vi "Calculate conductance ITX.vi"(0 "File or Folder Path":path=path "P:/expt/Leiden MNK/SA02836H.20170110/47", 5 "single ended?":bool=TRUE, 7 "index":T2={"N1"=18, "N2"=19, "N3"=4, "N4"=5, "V1"=8, "V2"=10, "V3"=10, "V4"=13, "CURRENT"=12, "Vsg"=1}, 9 "offset":i32, 11 "length":i32=1000) -> (3 "N Array":T1(array[cluster])=[{"N1"=191.996, "N2"=144.795, "N3"=0.00010057503022848991, "N4"=-1.0338940453395174e-05}, {"N1"=191.996, "N2"=147.003, "N3"=0.00010066534958225373, "N4"=-1.0380780420219314e-05}, {"N1"=191.996, "N2"=149.362, "N3"=0.00010045742974572892, "N4"=-1.0407899416737152e-05}, {"N1"=191.996, "N2"=151.724, "N3"=0.0001005426468584359, "N4"=-1.041982763249689e-05}, {"N1"=191.996, "N2"=154.337, "N3"=0.00010054163078601866, "N4"=-1.0324258520933678e-05}, {"N1"=191.996, "N2"=156.886, "N3"=0.00010056662242594223, "N4"=-1.038386753752895e-05}, {"N1"=191.996, "N2"=159.496, "N3"=0.0001006132221954114, "N4"=-1.0237620457409125e-05}, {"N1"=191.996, "N2"=161.991, "N3"=0.00010051966642671815, "N4"=-1.0219524315805733e-05}, {"N1"=191.996, "N2"=164.35, "N3"=0.00010054011068586918, "N4"=-1.0306705331260904e-05}, {"N1"=191.996, "N2"=166.841, "N3"=0.00010064457917184225, "N4"=-1.0165964089479782e-05}, {"N1"=191.996, "N2"=169.349, "N3"=0.00010053072958605225, "N4"=-1.0410678322353806e-05}, {"N1"=191.996, "N2"=172.005, "N3"=0.0001004938480593684, "N4"=-1.0388414744068434e-05}, {"N1"=191.996, "N2"=174.505, "N3"=0.00010066827534930882, "N4"=-1.0395636867591871e-05}, {"N1"=191.996, "N2"=177.006, "N3"=0.0001005048646735938, "N4"=-1.0223947706368497e-05}, {"N1"=191.996, "N2"=179.504, "N3"=0.00010058085140214634, "N4"=-1.0431970547534671e-05}, {"N1"=191.996, "N2"=181.84, "N3"=0.00010052922489490765, "N4"=-1.0355084186355676e-05}, {"N1"=191.996, "N2"=184.374, "N3"=0.00010058119857393249, "N4"=-1.0414147914325042e-05}, {"N1"=191.996, "N2"=187.017, "N3"=0.00010055623762781604, "N4"=-1.0471997511387608e-05}, {"N1"=191.996, "N2"=189.493, "N3"=0.00010061746471290358, "N4"=-1.0469366265831165e-05}, {"N1"=191.996, "N2"=192.044, "N3"=0.00010054215797227613, "N4"=-1.035195576109068e-05}, {"N1"=191.996, "N2"=194.506, "N3"=0.00010070522372706563, "N4"=-1.0337727806851342e-05}, {"N1"=191.996, "N2"=196.968, "N3"=0.00010065305882857154, "N4"=-1.0272321635940252e-05}, {"N1"=191.996, "N2"=199.515, "N3"=0.00010065777271444059, "N4"=-1.0350588285323707e-05}, {"N1"=191.996, "N2"=201.997, "N3"=0.00010058385854993672, "N4"=-1.0306678170450834e-05}, {"N1"=191.996, "N2"=204.265, "N3"=0.00010061221693842934, "N4"=-1.0065603355709244e-05}, {"N1"=191.996, "N2"=206.999, "N3"=0.0001005875811108127, "N4"=-1.0206305681344109e-05}, {"N1"=191.996, "N2"=209.539, "N3"=0.00010058820923197684, "N4"=-1.0493263333126373e-05}, {"N1"=191.996, "N2"=212.028, "N3"=0.00010061805295099033, "N4"=-1.0298862286088797e-05}, {"N1"=191.996, "N2"=214.443, "N3"=0.00010055810354804531, "N4"=-1.0563400445389847e-05}, {"N1"=191.996, "N2"=216.725, "N3"=0.00010053926676591393, "N4"=-1.038753898763444e-05}, {"N1"=191.996, "N2"=219.47, "N3"=0.00010058066546024038, "N4"=-1.03096656971029e-05}, {"N1"=191.996, "N2"=221.797, "N3"=0.000100521698263223, "N4"=-1.033180469731966e-05}, {"N1"=191.996, "N2"=224.497, "N3"=0.0001004795934350268, "N4"=-1.0405173181004657e-05}, {"N1"=191.996, "N2"=226.998, "N3"=0.00010059015791575789, "N4"=-1.033766826105032e-05}, {"N1"=191.996, "N2"=229.436, "N3"=0.00010060923714347418, "N4"=-1.0267885998498252e-05}, {"N1"=191.996, "N2"=231.634, "N3"=0.00010049651116289272, "N4"=-1.0430449385843277e-05}, {"N1"=191.996, "N2"=234.5, "N3"=0.00010055712089386373, "N4"=-1.0358131509413556e-05}, {"N1"=191.996, "N2"=236.999, "N3"=0.00010068379827598355, "N4"=-1.0302561579314388e-05}, {"N1"=191.996, "N2"=239.477, "N3"=0.00010047866336560874, "N4"=-1.0411909259862328e-05}, {"N1"=191.996, "N2"=241.853, "N3"=0.00010055343454259429, "N4"=-1.0243657310468301e-05}, {"N1"=191.996, "N2"=244.405, "N3"=0.00010058417717772568, "N4"=-1.0269493681777803e-05}, {"N1"=191.996, "N2"=246.91, "N3"=0.00010062819456533582, "N4"=-1.0272141148598907e-05}, {"N1"=191.996, "N2"=249.488, "N3"=0.00010056821029236928, "N4"=-1.0340020021854818e-05}, {"N1"=191.996, "N2"=251.704, "N3"=0.00010065759557074449, "N4"=-1.0329641383071122e-05}, {"N1"=191.996, "N2"=254.492, "N3"=0.00010057796952190451, "N4"=-1.0284612827778078e-05}, {"N1"=191.996, "N2"=256.799, "N3"=0.00010063577042569525, "N4"=-1.0329227866710886e-05}, {"N1"=189.506, "N2"=256.99, "N3"=0.00010053195853199196, "N4"=-1.0445442874501309e-05}, {"N1"=189.506, "N2"=254.642, "N3"=0.00010062373739047002, "N4"=-1.038267676413735e-05}, {"N1"=189.506, "N2"=252.252, "N3"=0.00010060901043629462, "N4"=-1.0423317753346132e-05}, {"N1"=189.506, "N2"=249.855, "N3"=0.00010050094587740504, "N4"=-1.0431223967160507e-05}, {"N1"=189.506, "N2"=246.999, "N3"=0.00010058974428219982, "N4"=-1.0340299277280957e-05}, {"N1"=189.506, "N2"=244.524, "N3"=0.00010055656468780623, "N4"=-1.053351676682195e-05}, {"N1"=189.506, "N2"=242.248, "N3"=0.00010055388255591169, "N4"=-1.0216325327280904e-05}, {"N1"=189.506, "N2"=240.113, "N3"=0.00010057451174382039, "N4"=-1.041060384291682e-05}, {"N1"=189.506, "N2"=236.998, "N3"=0.00010054319017101952, "N4"=-1.0348870506195839e-05}, {"N1"=189.506, "N2"=234.866, "N3"=0.00010050860466242158, "N4"=-1.0475965819222953e-05}, {"N1"=189.506, "N2"=231.979, "N3"=0.00010060735713010531, "N4"=-1.0374517256243438e-05}, {"N1"=189.506, "N2"=229.88, "N3"=0.00010049947613491992, "N4"=-1.0491154630192516e-05}, {"N1"=189.506, "N2"=227.267, "N3"=0.00010062560576095063, "N4"=-1.0555557528305423e-05}, {"N1"=189.506, "N2"=224.473, "N3"=0.00010054870210895435, "N4"=-1.0387256544361327e-05}, {"N1"=189.506, "N2"=222.338, "N3"=0.0001005705880949266, "N4"=-1.0359666369953541e-05}, {"N1"=189.506, "N2"=219.943, "N3"=0.00010052399645025834, "N4"=-1.0310144901537403e-05}, {"N1"=189.506, "N2"=217.359, "N3"=0.00010060901318214533, "N4"=-1.0430222257765288e-05}, {"N1"=189.506, "N2"=214.968, "N3"=0.0001005359008706473, "N4"=-1.0310194088582675e-05}, {"N1"=189.506, "N2"=212.385, "N3"=0.00010054874079276358, "N4"=-1.0350840870693861e-05}, {"N1"=189.506, "N2"=209.538, "N3"=0.00010052877064697572, "N4"=-1.0448750460944099e-05}, {"N1"=189.506, "N2"=207.267, "N3"=0.00010053680956204742, "N4"=-1.0355852855433731e-05}, {"N1"=189.506, "N2"=204.668, "N3"=0.00010057308714312922, "N4"=-1.0381850165958104e-05}, {"N1"=189.506, "N2"=201.992, "N3"=0.00010051465119619463, "N4"=-1.0253710037528991e-05}, {"N1"=189.506, "N2"=199.708, "N3"=0.00010054552600488515, "N4"=-1.0111514624342852e-05}, {"N1"=189.506, "N2"=197.028, "N3"=0.00010056463679786198, "N4"=-1.0131100186631911e-05}, {"N1"=189.506, "N2"=194.795, "N3"=0.00010052779216466223, "N4"=-1.0611826314801406e-05}, {"N1"=189.506, "N2"=192.336, "N3"=0.00010061170953168135, "N4"=-1.0313720182691726e-05}, {"N1"=189.506, "N2"=189.856, "N3"=0.00010049183044402859, "N4"=-1.0574827403736794e-05}, {"N1"=189.506, "N2"=187.38, "N3"=0.00010057831497383143, "N4"=-1.0526665896714861e-05}, {"N1"=189.506, "N2"=184.506, "N3"=0.0001005504195817918, "N4"=-1.0419727243247705e-05}, {"N1"=189.506, "N2"=182.041, "N3"=0.00010053309735838938, "N4"=-1.027504174089921e-05}, {"N1"=189.506, "N2"=179.521, "N3"=0.00010063619607854753, "N4"=-1.0259288158518756e-05}, {"N1"=189.506, "N2"=177.348, "N3"=0.00010056552179621183, "N4"=-1.0306944055227605e-05}, {"N1"=189.506, "N2"=174.768, "N3"=0.00010050767014227269, "N4"=-1.0363158516396958e-05}, {"N1"=189.506, "N2"=171.99, "N3"=0.00010049993887402406, "N4"=-1.0288583567424436e-05}], 4 "A vs D":cluster{dbl[], dbl[]}[](graph), 6 "Index, Wavenames":string[][](table)=[["0", "'time.SA02836H.20170110.000034'\n"], ["1", "'Vsg.SA02836H.20170110.000034'\n"], ["2", "'T.SA02836H.20170110.000034'\n"], ["3", "'B.SA02836H.20170110.000034'\n"], ["4", "'X0.SA02836H.20170110.000034'\n"], ["5", "'Y0.SA02836H.20170110.000034'\n"], ["6", "'X1.SA02836H.20170110.000034'\n"], ["7", "'Y1.SA02836H.20170110.000034'\n"], ["8", "'X2.SA02836H.20170110.000034'\n"], ["9", "'Y2.SA02836H.20170110.000034'\n"], ["10", "'X3.SA02836H.20170110.000034'\n"], ["11", "'Y3.SA02836H.20170110.000034'\n"], ["12", "'X4.SA02836H.20170110.000034'\n"], ["13", "'Y4.SA02836H.20170110.000034'\n"], ["14", "'X5.SA02836H.20170110.000034'\n"], ["15", "'Y5.SA02836H.20170110.000034'\n"], ["16", "'B_rate.SA02836H.20170110.000034'\n"], ["17", "'R4t(e2/h).SA02836H.20170110.000034'\n"], ["18", "'axis1.SA02836H.20170110.000034'\n"], ["19", "'axis2.SA02836H.20170110.000034'\n"], ["", ""]], 8 "Comments":string="IGOR\nX// Date: 2/20/2017 3:49 PM\nX// B=18T\nX// large axis: 192 -- 184.5, 2.5 deg steps\nX// small axis: 144.5 -- 257, 2.5 deg steps\nX// sweep Vsg: 50mV to 170mV, 250uV steps\nX// Vbg=0.45V\nX// T<50mK\nX// \nX// lockin settings: \nX// tc=0.3s\nX// order=4\nX// prefilters OFF\nX// \nX// 0: 1, voltage\nX// 1: 2, current, 100uV AC 240uV DC, 13 Hz\nX// 2: 3, voltage\nX// 3: 4, voltage\nX// 4: 5, current\nX// 5: 7, voltage\nX//  \nX// KH gain=100x, shunt resistor=50kOhm\nX// \nX// axis1=189.506000\nX// axis2=171.990000\n\n\n\n\n\n\n\n\n\n\n\n\n\n\n\n\n\n\n\n\n\n\n\n\n\n\n\n\n\n\n\n\n\n\n\n\n\n\n\n\n\n\nX \nX Display/R 'time.SA02836H.20170110.000034'\nX AppendToGraph 'Vsg.SA02836H.20170110.000034'\nX AppendToGraph 'T.SA02836H.20170110.000034'\nX AppendToGraph 'B.SA02836H.20170110.000034'\nX AppendToGraph 'X0.SA02836H.20170110.000034'\nX AppendToGraph 'Y0.SA02836H.20170110.000034'\nX AppendToGraph 'X1.SA02836H.20170110.000034'\nX AppendToGraph 'Y1.SA02836H.20170110.000034'\nX AppendToGraph 'X2.SA02836H.20170110.000034'\nX AppendToGraph 'Y2.SA02836H.20170110.000034'\nX AppendToGraph 'X3.SA02836H.20170110.000034'\nX AppendToGraph 'Y3.SA02836H.20170110.000034'\nX AppendToGraph 'X4.SA02836H.20170110.000034'\nX AppendToGraph 'Y4.SA02836H.20170110.000034'\nX AppendToGraph 'X5.SA02836H.20170110.000034'\nX AppendToGraph 'Y5.SA02836H.20170110.000034'\nX AppendToGraph 'B_rate.SA02836H.20170110.000034'\nX AppendToGraph 'R4t(e2/h).SA02836H.20170110.000034'\nX AppendToGraph 'axis1.SA02836H.20170110.000034'\nX AppendToGraph 'axis2.SA02836H.20170110.000034'\nX Label bottom \"x label\"\nX Label left \"y label\"\nX ModifyGraph rgb('time.SA02836H.20170110.000034')=(65280,0,0)\nX ModifyGraph rgb('Vsg.SA02836H.20170110.000034')=(65280,18432,0)\nX ModifyGraph rgb('T.SA02836H.20170110.000034')=(65280,35328,0)\nX ModifyGraph rgb('B.SA02836H.20170110.000034')=(65280,52224,0)\nX ModifyGraph rgb('X0.SA02836H.20170110.000034')=(60416,65280,0)\nX ModifyGraph rgb('Y0.SA02836H.20170110.000034')=(41984,65280,0)\nX ModifyGraph rgb('X1.SA02836H.20170110.000034')=(25088,65280,0)\nX ModifyGraph rgb('Y1.SA02836H.20170110.000034')=(8192,65280,0)\nX ModifyGraph rgb('X2.SA02836H.20170110.000034')=(0,65280,10240)\nX ModifyGraph rgb('Y2.SA02836H.20170110.000034')=(0,65280,28672)\nX ModifyGraph rgb('X3.SA02836H.20170110.000034')=(0,65280,45568)\nX ModifyGraph rgb('Y3.SA02836H.20170110.000034')=(0,65280,62464)\nX ModifyGraph rgb('X4.SA02836H.20170110.000034')=(0,50176,65280)\nX ModifyGraph rgb('Y4.SA02836H.20170110.000034')=(0,31744,65280)\nX ModifyGraph rgb('X5.SA02836H.20170110.000034')=(0,14848,65280)\nX ModifyGraph rgb('Y5.SA02836H.20170110.000034')=(2048,0,65280)\nX ModifyGraph rgb('B_rate.SA02836H.20170110.000034')=(20480,0,65280)\nX ModifyGraph rgb('R4t(e2/h).SA02836H.20170110.000034')=(38912,0,65280)\nX ModifyGraph rgb('axis1.SA02836H.20170110.000034')=(55808,0,65280)\nX ModifyGraph rgb('axis2.SA02836H.20170110.000034')=(65280,0,58368)\nX Legend/C/N=text0/J \"\\\\s('time.SA02836H.20170110.000034') time\\r\\\\s('Vsg.SA02836H.20170110.000034') Vsg\\r\\\\s('T.SA02836H.20170110.000034') T\\r\\\\s('B.SA02836H.20170110.000034') B\\r\\\\s('X0.SA02836H.20170110.000034') X0\\r\\\\s('Y0.SA02836H.20170110.000034') Y0\\r\\\\s('X1.SA02836H.20170110.000034') X1\\r\\\\s('Y1.SA02836H.20170110.000034') Y1\\r\\\\s('X2.SA02836H.20170110.000034') X2\\r\\\\s('Y2.SA02836H.20170110.000034') Y2\\r\\\\s('X3.SA02836H.20170110.000034') X3\\r\\\\s('Y3.SA02836H.20170110.000034') Y3\\r\\\\s('X4.SA02836H.20170110.000034') X4\\r\\\\s('Y4.SA02836H.20170110.000034') Y4\\r\\\\s('X5.SA02836H.20170110.000034') X5\\r\\\\s('Y5.SA02836H.20170110.000034') Y5\\r\\\\s('B_rate.SA02836H.20170110.000034') B_rate\\r\\\\s('R4t(e2/h).SA02836H.20170110.000034') R4t (e2/h)\\r\\\\s('axis1.SA02836H.20170110.000034') axis 1\\r\\\\s('axis2.SA02836H.20170110.000034') axis 2\"\nX ModifyGraph mirror(bottom)=1\nX ModifyGraph width=216\nX ModifyGraph height={Aspect,0.6}\nX ModifyGraph Log(bottom)=0\nX ModifyGraph Log(left)=0\nX \n")   [LabVIEW 2016]
uses:
  <vilib>/Utility/miscctls.llb/LVOffsetAndMultiplierTypeDef.ctl
  <vilib>/Analysis/NI_AALPro.lvlib
panel:
  out "A vs D diff":cluster{dbl[], dbl[]}[](graph)
  in  "Numeric":dbl=50.0
  in  "dy/dx vs x":bool=TRUE
  out "angle phi":dbl[](array[numeric])=[90.00000409114715, 90.00000404600523, 90.0000039925062, 90.00000393485637, 90.00000383275845, 90.00000379225543, 90.00000367766242, 90.00000361461817, 90.00000359312878, 90.00000349114927, 90.00000352224065, 90.00000346043615, 90.00000341323239, 90.00000330943048, 90.00000332977474, 90.00000326277288, 90.00000323628453, 90.00000320827124, 90.00000316555494, 90.00000308847648, 90.0000030451923, 90.00000298810302, 90.00000297243328, 90.0000029234551, 90.00000282337449, 90.0000028250293, 90.00000286924964, 90.00000278303499, 90.0000028223736, 90.00000274616285, 90.00000269148555, 90.00000266896669, 90.00000265559233, 90.00000260929507, 90.00000256414222, 90.00000258002162, 90.0000025308197, 90.00000249069954, 90.00000249108874, 90.00000242675647, 90.00000240747384, 90.00000238366341, 90.00000237462126, 90.00000235135259, 90.00000231545553, 90.00000230460853, 90.00000232880578, 90.00000233615648, 90.00000236752183, 90.00000239204782, 90.00000239861501, 90.00000246816694, 90.00000241633502, 90.00000248417896, 90.00000250190551, 90.00000255562162, 90.0000025623701, 90.00000261483767, 90.00000266113821, 90.0000026513031, 90.00000266965233, 90.00000268582218, 90.00000274940405, 90.00000274799322, 90.00000279237939, 90.0000028570918, 90.0000028627165, 90.00000290634686, 90.00000290850286, 90.00000290097098, 90.00000294612585, 90.00000312129605, 90.00000307239746, 90.00000319132911, 90.00000321877216, 90.0000032357018, 90.00000323397765, 90.00000327434626, 90.00000332986215, 90.00000339744831, 90.00000342748076]
  in  "e^2/h?":bool=TRUE
  in  "T=conductance\nF=resistance":bool=TRUE
  out "angle theta":dbl[](array[numeric])=[3.979781592245742e-05, 3.923525148650886e-05, 3.8535817310704016e-05, 3.7968082347300365e-05, 3.7324887158624575e-05, 3.6727579420033637e-05, 3.614330763786105e-05, 3.5553534729170675e-05, 3.505034386417848e-05, 3.456290490596515e-05, 3.401252157763598e-05, 3.347503480032623e-05, 3.3052733780554244e-05, 3.253282129605657e-05, 3.210434466738831e-05, 3.1675650595023693e-05, 3.1256457942296714e-05, 3.080708181495749e-05, 3.04230555923191e-05, 2.9996465991900285e-05, 2.9664813910527506e-05, 2.9278844614143605e-05, 2.8906425841285385e-05, 2.85302780835941e-05, 2.8221454473483897e-05, 2.7841892323532745e-05, 2.7504568876298417e-05, 2.7189756904348253e-05, 2.6867535564891757e-05, 2.657965468232256e-05, 2.6258019918388047e-05, 2.596729919687742e-05, 2.5644247500042603e-05, 2.5389613605084715e-05, 2.512458667494002e-05, 2.4858293451836762e-05, 2.4569290521129328e-05, 2.4340848301301122e-05, 2.403990087551123e-05, 2.3821442838564363e-05, 2.3579913823692036e-05, 2.3350900524947192e-05, 2.3095836284456867e-05, 2.2912847639044594e-05, 2.2643906942458915e-05, 2.2453377596639828e-05, 2.2413545002011955e-05, 2.264086628013591e-05, 2.2852035579448446e-05, 2.3046487105912263e-05, 2.33335673815276e-05, 2.3561968391426693e-05, 2.378270649956887e-05, 2.3999096465037315e-05, 2.430695809914132e-05, 2.4519167746311992e-05, 2.4848701613163618e-05, 2.5048702913721435e-05, 2.5368498378776492e-05, 2.5664629003759286e-05, 2.5916713476722578e-05, 2.6186788105952318e-05, 2.652051139503117e-05, 2.67960013091869e-05, 2.7125354816864744e-05, 2.7488447335136823e-05, 2.7791857235427556e-05, 2.8154931039059754e-05, 2.8511353384149216e-05, 2.8846287024066625e-05, 2.9244215323624077e-05, 2.9568614260134713e-05, 2.997164506780307e-05, 3.032697286357333e-05, 3.0754151769332044e-05, 3.1224538336453484e-05, 3.164189484793498e-05, 3.211896826305098e-05, 3.248968109847988e-05, 3.2950341640601424e-05, 3.3479983364170464e-05]
  in  "log scale?":bool
  in  "calculate Ey":bool=TRUE
  in  "background":enum16{"do nothing", "subtract", "divide"}(ring)
  in  "Background":cluster{dbl[], dbl[]}[](graph)
  in  "A offset":dbl format="%#_6p"
  out "E 2":dbl[][](graph)
  out "counter":i32=80
  out "Path":path=path "P:/expt/Leiden MNK/SA02836H.20170110/47/47 - Sweep axis 1,2 - 1/SA02836H.20170110.000034.itx"
  in  "file contains 2D data?":bool
  out "N":cluster{"N1":dbl, "N2":dbl, "N3":dbl, "N4":dbl}={"N1"=189.506, "N2"=171.99, "N3"=0.00010049993887402406, "N4"=-1.0288583567424436e-05} {"N4" format="%#_6p"; "N3" format="%#_6p"; "N2" format="%#_6p"; "N1" format="%#_20p"}
  in  "Ey":T3={"Offset"=0.0, "Multiplier"=1.0}
  in  "Ex":T3={"Offset"=0.0, "Multiplier"=1.0}
  in  "recolor traces?":bool
  out "C vs D":cluster{dbl[], dbl[]}[](graph)
  out "E":dbl[][](graph)
  in  "B x name":string="Vsg (V)"
  in  "A y name":string="Conductance (S)"
  in  "Ex name":string="Ex name"
  in  "Ez name":string="Ez name"
  in  "D x name":string="Vsg (V)"
  in  "C y name":string="Conductance (S)"
  in  "Ey name":string="Ey name"
  out "time":string[][](table)=[["2/19/2017", "7:43 PM"], ["2/19/2017", "7:56 PM"], ["2/19/2017", "8:09 PM"], ["2/19/2017", "8:22 PM"], ["2/19/2017", "8:34 PM"], ["2/19/2017", "8:47 PM"], ["2/19/2017", "9:01 PM"], ["2/19/2017", "9:15 PM"], ["2/19/2017", "9:28 PM"], ["2/19/2017", "9:40 PM"], ["2/19/2017", "9:52 PM"], ["2/19/2017", "10:05 PM"], ["2/19/2017", "10:19 PM"], ["2/19/2017", "10:33 PM"], ["2/19/2017", "10:49 PM"], ["2/19/2017", "11:02 PM"], ["2/19/2017", "11:15 PM"], ["2/19/2017", "11:29 PM"], ["2/19/2017", "11:42 PM"], ["2/19/2017", "11:57 PM"], ["2/20/2017", "12:11 AM"], ["2/20/2017", "12:25 AM"], ["2/20/2017", "12:41 AM"], ["2/20/2017", "12:55 AM"], ["2/20/2017", "1:08 AM"], ["2/20/2017", "1:22 AM"], ["2/20/2017", "1:36 AM"], ["2/20/2017", "1:50 AM"], ["2/20/2017", "2:03 AM"], ["2/20/2017", "2:16 AM"], ["2/20/2017", "2:33 AM"], ["2/20/2017", "2:46 AM"], ["2/20/2017", "3:01 AM"], ["2/20/2017", "3:22 AM"], ["2/20/2017", "5:13 AM"], ["2/20/2017", "5:25 AM"], ["2/20/2017", "5:38 AM"], ["2/20/2017", "6:10 AM"], ["2/20/2017", "6:22 AM"], ["2/20/2017", "6:35 AM"], ["2/20/2017", "6:47 AM"], ["2/20/2017", "7:00 AM"], ["2/20/2017", "7:13 AM"], ["2/20/2017", "7:26 AM"], ["2/20/2017", "7:39 AM"], ["2/20/2017", "7:51 AM"], ["2/20/2017", "8:09 AM"], ["2/20/2017", "8:22 AM"], ["2/20/2017", "8:35 AM"], ["2/20/2017", "8:48 AM"], ["2/20/2017", "9:01 AM"], ["2/20/2017", "9:14 AM"], ["2/20/2017", "9:27 AM"], ["2/20/2017", "9:40 AM"], ["2/20/2017", "9:57 AM"], ["2/20/2017", "10:10 AM"], ["2/20/2017", "10:24 AM"], ["2/20/2017", "10:37 AM"], ["2/20/2017", "10:50 AM"], ["2/20/2017", "11:08 AM"], ["2/20/2017", "11:21 AM"], ["2/20/2017", "11:35 AM"], ["2/20/2017", "11:48 AM"], ["2/20/2017", "12:01 PM"], ["2/20/2017", "12:15 PM"], ["2/20/2017", "12:29 PM"], ["2/20/2017", "12:42 PM"], ["2/20/2017", "12:55 PM"], ["2/20/2017", "1:09 PM"], ["2/20/2017", "1:21 PM"], ["2/20/2017", "1:37 PM"], ["2/20/2017", "1:50 PM"], ["2/20/2017", "2:03 PM"], ["2/20/2017", "2:16 PM"], ["2/20/2017", "2:29 PM"], ["2/20/2017", "2:43 PM"], ["2/20/2017", "2:56 PM"], ["2/20/2017", "3:10 PM"], ["2/20/2017", "3:23 PM"], ["2/20/2017", "3:36 PM"], ["2/20/2017", "3:49 PM"]]
  in  "B is time?":bool
  in  "D  is time?":bool
  in  "Generate Folder Index File?":bool
  in  "pattern":string="*.itx"
  in  "Use Folder Index File?":bool
  # "CURRENT/(V1-V2)"
  # "CURRENT/(V3-V4)"
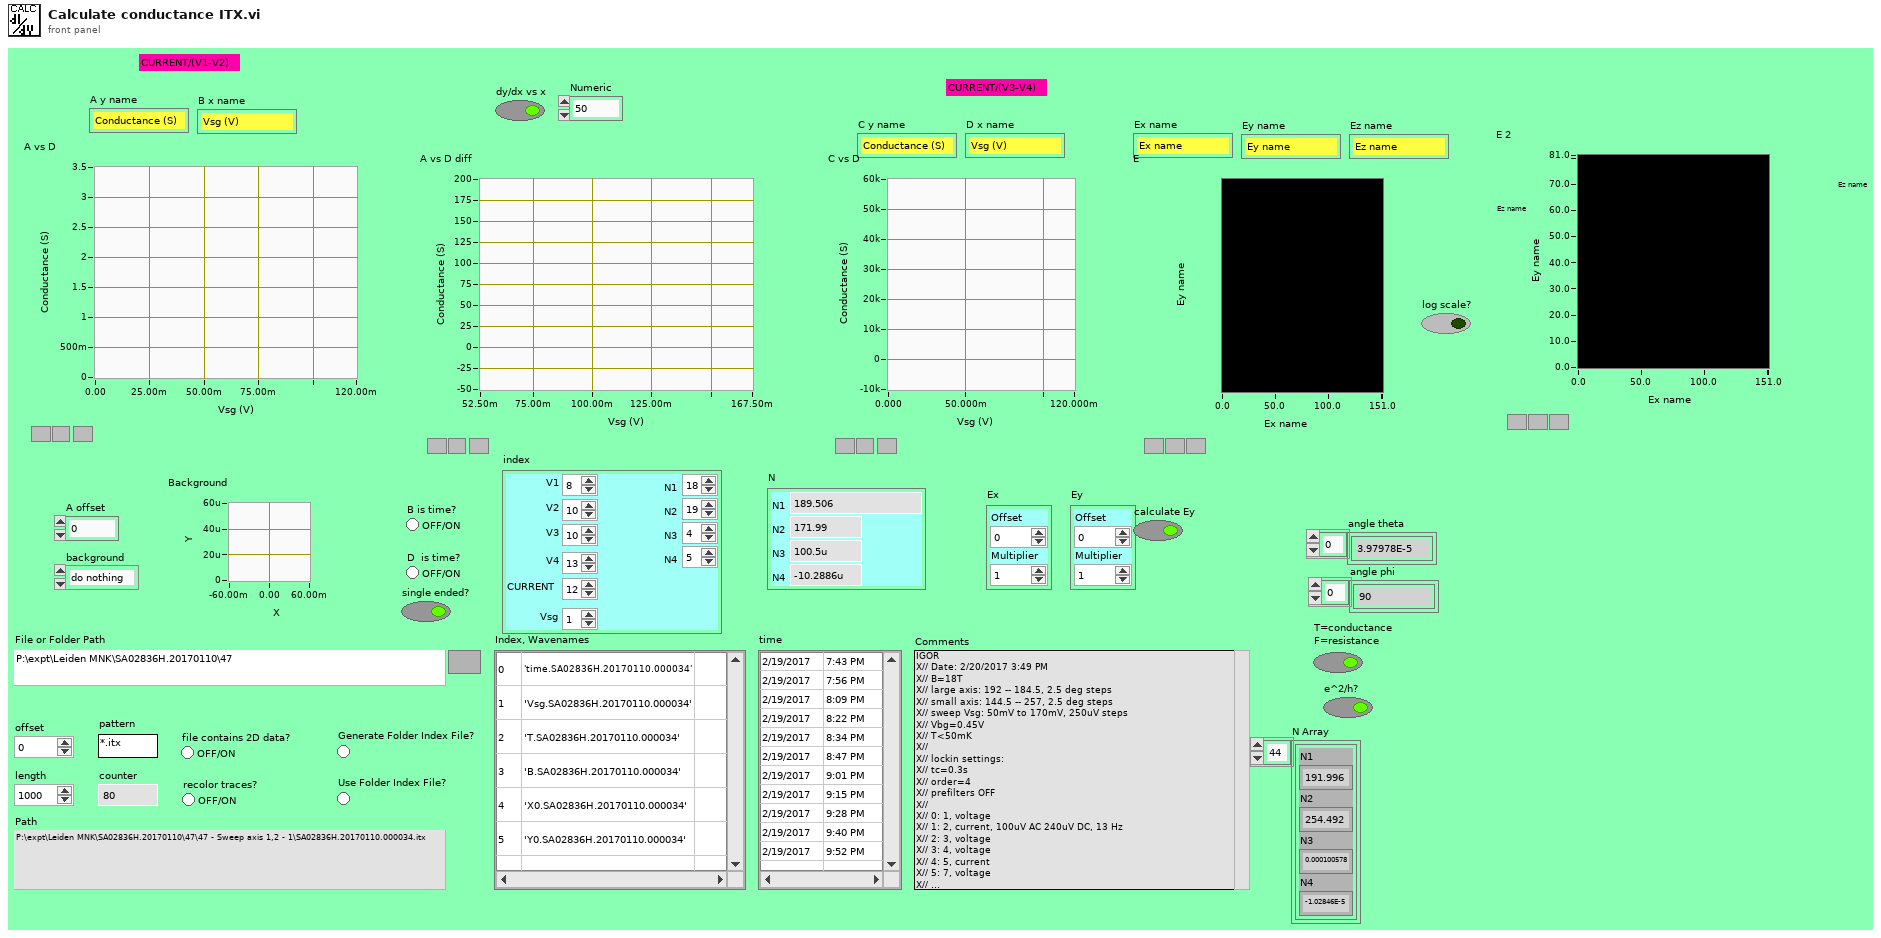
[diagram p1: front panel]
types:
  T1 = cluster{"N1":dbl, "N2":dbl, "N3":dbl, "N4":dbl}[]
  T2 = cluster{"N1":i32, "N2":i32, "N3":i32, "N4":i32, "V1":i32, "V2":i32, "V3":i32, "V4":i32, "CURRENT":i32, "Vsg":i32}
  T3 = typedef "LVOffsetAndMultiplierTypeDef.ctl" = cluster{"Offset":dbl, "Multiplier":dbl}
  T4 = cluster{"Decimated Array":dbl[], "Decimated Array":dbl[]}
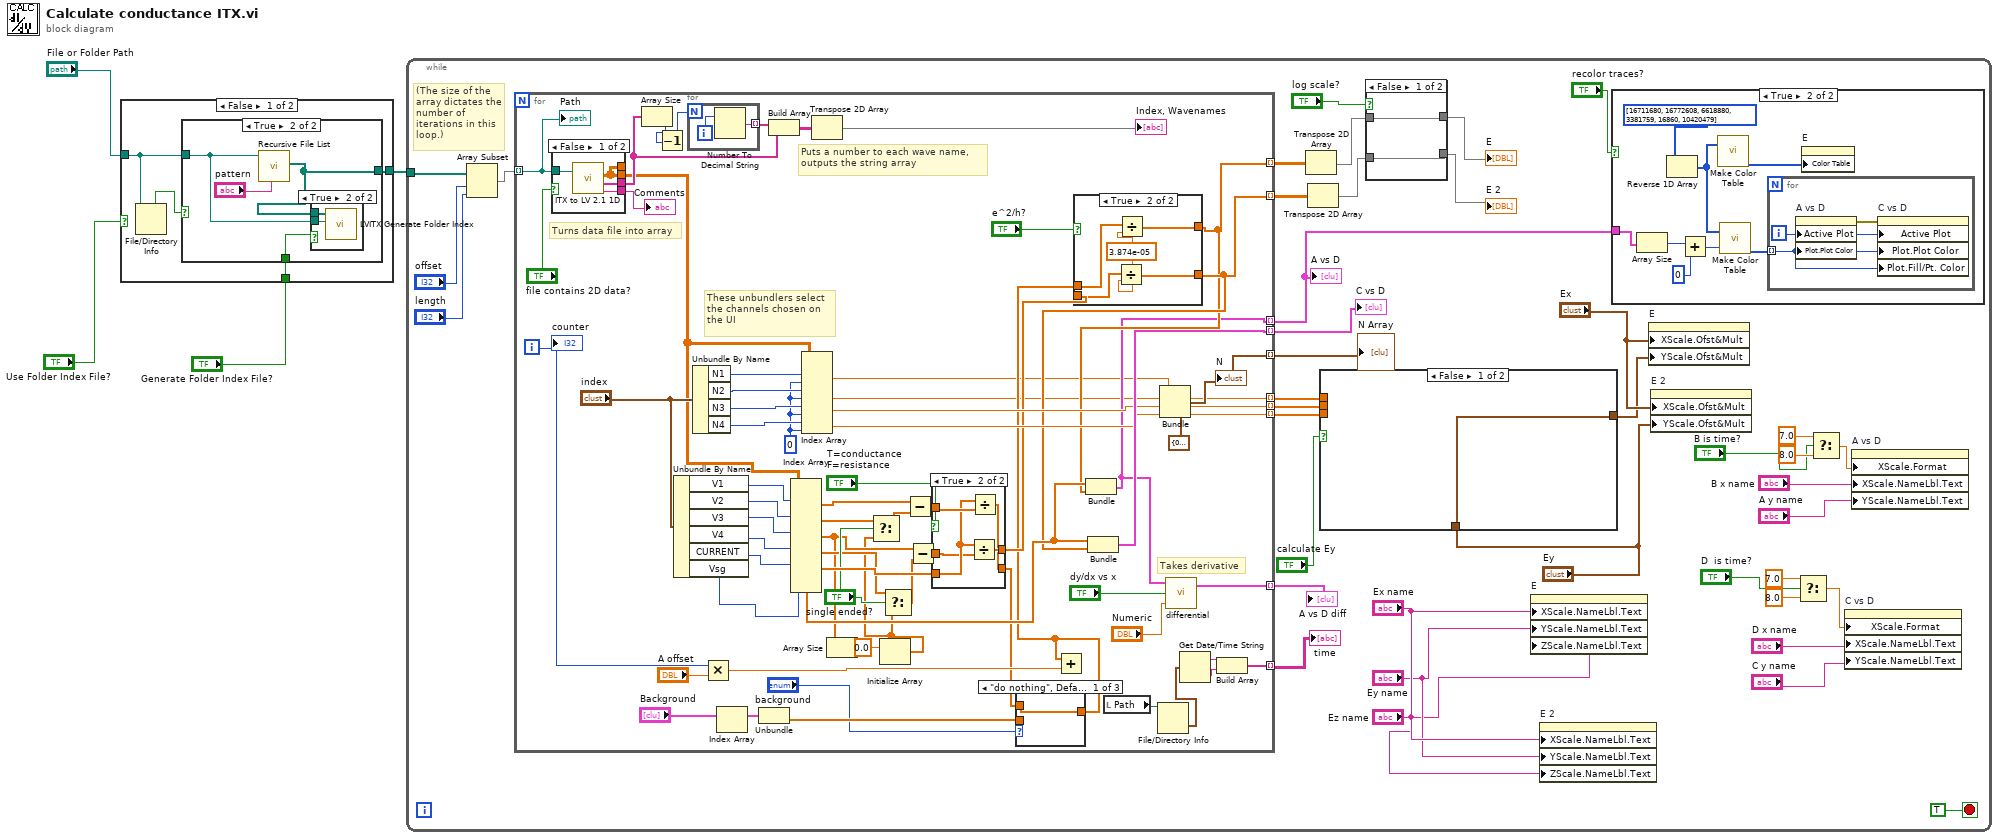
[diagram p0: block diagram]
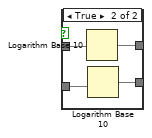
[diagram p2: hidden frame]
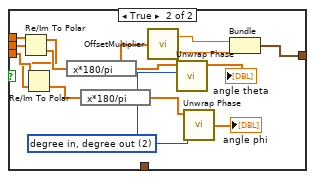
[diagram p3: hidden frame]
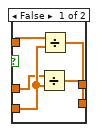
[diagram p6: hidden frame]
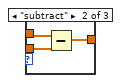
[diagram p7: hidden frame]
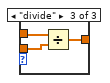
[diagram p8: hidden frame]
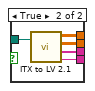
[diagram p9: hidden frame]
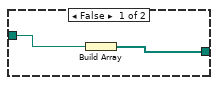
[diagram p10: hidden frame]
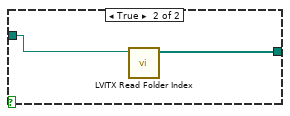
[diagram p12: hidden frame]
diagram:
  n1 = case shown="False" "Use Folder Index File?" {
    tunnel: [w6 w17] -> w2
    tunnel: "File or Folder Path" -> [w8 w18]
    tunnel: "Generate Folder Index File?" -> [w5 _]
    frame False {
      n2 = File/Directory Info(path=w8) -> (directory=w7:bool)  [unwired: 1 in, 6 out]
      n3 = case shown="True" w7 {
        tunnel: [w10 w13] -> w6
        tunnel: w8 -> [w9 w12]
        tunnel: w5 -> [_ w11]
        frame False {
          n4 = Build Array(w9) -> (w10:path[])
        }
        frame True {
          n5 = call <vilib>:"Recursive File List.vi"("pattern"="pattern", "Folder Path"=w12) -> ("All Files in Dir"=w13:path[])  [unwired: 5 in, 4 out]
          n6 = case shown="True" w11 {
            tunnel: w13 -> [_ w16]
            tunnel: w12 -> [_ w15]
            frame False {
            }
            frame True {
              n7 = call <userlib>:"LVITX Generate Folder Index.vi"("File or Folder Path"=w15, "All Files in Dir"=w16) -> ()  [unwired: 10 in]
            }
          }
        }
      }
    }
    frame True {
      n8 = call <userlib>:"LVITX Read Folder Index.vi"("File or Folder Path"=w18) -> ("Array"=w17:path[])  [unwired: 10 in]
    }
  }
  n9 = while {
    tunnel: w2 -> [w50]
    stop <- TRUE stop-if-true
    # "(The size of the array dictates the number of\niterations in this loop.)"
    n10 = Array Subset(array=w50, index="offset", length="length") -> (w49:path[])
    n11 = for {
      tunnel: w49 -> [w156] mode=indexing
      tunnel: [w156] -> _ mode=indexing
      tunnel: [w139] -> w53 mode=indexing
      tunnel: [w97] -> w39 mode=indexing
      tunnel: [w126] -> w40 mode=indexing
      tunnel: [w108] -> w38 mode=indexing
      tunnel: [w109] -> w37 mode=indexing
      tunnel: [w91] -> w31 mode=indexing
      tunnel: [w115] -> w30 mode=indexing
      tunnel: [w114] -> w29 mode=indexing
      tunnel: [w107] -> w20 mode=indexing
      tunnel: [w94] -> w19 mode=indexing
      i -> [w123]
      w137 = 0 ("disabled index (col)")
      # "Takes derivative"
      # "These unbundlers select\nthe channels chosen on\nthe UI"
      # "Puts a number to each wave name,\noutputs the string array"
      # "Turns data file into array"
      n12 = case shown="False" "file contains 2D data?" {
        tunnel: [w186 w189] -> w93
        tunnel: [w184 w190] -> w131
        tunnel: w156 -> [w185 w191]
        tunnel: [w183 w188] -> w149
        tunnel: [w184 w187] -> _
        frame False {
          n13 = call <userlib>:"ITX to LV 2.1 1D.vi"("file (use dialog)"=w185) -> ("1D arrays"=w184:dbl[][], "wave names"=w183:string[], "Notes"=w186:string)  [unwired: 2 in]
        }
        frame True {
          n14 = call <userlib>:"ITX to LV 2.1.vi"("file (use dialog)"=w191) -> ("2D array"=w187:dbl[][], "1D arrays"=w190:dbl[][], "wave names"=w188:string[], "Notes"=w189:string)  [unwired: 1 in]
        }
      }
      "Comments" <- w93
      n15 = Array Size(array=w149) -> (size(s)=w152:i32)
      n16 = Decrement(x=w152) -> (x-1=w151:i32)
      n17 = Unbundle By Name("index") -> ("V1"=w136:i32, "V2"=w135:i32, "V3"=w134:i32, "V4"=w133:i32, "CURRENT"=w130:i32, "Vsg"=w125:i32)
      n18 = for {
        N: w151 -> [_]
        tunnel: [w181] -> w154 mode=indexing
        i -> [w182]
        n19 = Number To Decimal String(number=w182) -> (decimal integer string=w181:string)  [unwired: 1 in]
      }
      n20 = Unbundle By Name("index") -> ("N1"=w144:i32, "N2"=w145:i32, "N3"=w146:i32, "N4"=w147:i32)
      n21 = Multiply(x=w123, y="A offset") -> (x*y=w121:dbl)
      n22 = Index Array(array="Background") -> (element=w117:cluster{dbl[], dbl[]})  [unwired: 1 in]
      n23 = Unbundle(w117) -> (w118:dbl[])  [unwired: 1 out]
      n24 = Build Array(w154, w149) -> (w150:string[][])
      n25 = Index Array(array=w131, index (row) #1=w136, index (row) #2=w135, index (row) #3=w134, index (row) #4=w133, index (row) #5=w130, index (row) #6=w125) -> (element #1=w132:dbl[], element #2=w105:dbl[], element #3=w101:dbl[], element #4=w103:dbl[], element #5=w128:dbl[], element #6=w124:dbl[])  [unwired: 6 in]
      n26 = Index Array(array=w131, index (row) #1=w144, index (col) #1=w137, index (row) #2=w145, index (col) #2=w137, index (row) #3=w146, index (col) #3=w137, index (row) #4=w147, index (col) #4=w137) -> (element #1=w92:dbl, element #2=w91:dbl, element #3=w115:dbl, element #4=w114:dbl)
      n27 = Transpose 2D Array(2D array=w150) -> (transposed array=→"Index, Wavenames":string[][])
      n28 = Array Size(array=w101) -> (size(s)=w99:i32)
      n29 = Initialize Array(0.0 ("element"), w99) -> (w98:dbl[])
      n30 = Select(t=w105, s="single ended?", f=w98) -> (s? t:f=w104:dbl[])
      n31 = Select(t=w103, s="single ended?", f=w98) -> (s? t:f=w102:dbl[])
      n32 = Subtract(x=w132, y=w104) -> (x-y=w129:dbl[])
      n33 = Subtract(x=w101, y=w102) -> (x-y=w127:dbl[])
      n34 = case shown="True" "T=conductance\nF=resistance" {
        tunnel: w129 -> [w168 w173]
        tunnel: w128 -> [w166 w172]
        tunnel: w127 -> [w165 w171]
        tunnel: [w164 w170] -> w112
        tunnel: [w167 w169] -> w120
        frame False {
          n35 = Divide(x=w165, y=w166) -> (x/y=w164:dbl[])
          n36 = Divide(x=w168, y=w166) -> (x/y=w167:dbl[])
        }
        frame True {
          n37 = Divide(x=w172, y=w171) -> (x/y=w170:dbl[])
          n38 = Divide(x=w172, y=w173) -> (x/y=w169:dbl[])
        }
      }
      n39 = case shown="\"do nothing\", Default" "background" {
        tunnel: w120 -> [w174 w177 w180]
        tunnel: [w174 w176 w178] -> w111
        tunnel: w118 -> [_ w175 w179]
        frame "do nothing", Default {
        }
        frame "subtract" {
          n40 = Subtract(x=w177, y=w175) -> (x-y=w176:dbl[])
        }
        frame "divide" {
          n41 = Divide(x=w180, y=w179) -> (x/y=w178:dbl[])
        }
      }
      n42 = Add(x=w111, y=w121) -> ()  [unwired: 1 out]
      n43 = case shown="True" "e^2/h?" {
        tunnel: w112 -> [w157 w161]
        tunnel: w111 -> [w158 w163]
        tunnel: [w158 w162] -> w108
        tunnel: [w157 w160] -> w109
        frame False {
        }
        frame True {
          w159 = 3.874e-05
          n44 = Divide(x=w161, y=w159) -> (x/y=w160:dbl[])
          n45 = Divide(x=w163, y=w159) -> (x/y=w162:dbl[])
        }
      }
      n46 = Bundle("1D arrays"=w124, w108) -> (w97:cluster{"1D arrays":dbl[], dbl[]})  [unwired: 1 in]
      n47 = Bundle("1D arrays"=w124, w109) -> (w126:cluster{"1D arrays":dbl[], dbl[]})  [unwired: 1 in]
      n48 = local read "Path"() -> (w143:path)
      n49 = File/Directory Info(path=w143) -> (last mod=w142:timestamp)  [unwired: 1 in, 6 out]
      n50 = Bundle(cluster=cluster{"N1":dbl, "N2":dbl, "N3":dbl, "N4":dbl} {"N1"=0.0, "N2"=0.0, "N3"=0.0, "N4"=0.0}, "N1"=w92, "N2"=w91, "N3"=w115, "N4"=w114) -> (w107:cluster{"N1":dbl, "N2":dbl, "N3":dbl, "N4":dbl})
      "N" <- w107
      n51 = call <userlib>:"differential.vi"("Numeric"="Numeric", "dy/dx vs x"="dy/dx vs x", "A vs B 2"=w97) -> ("A vs B 3"=w94:T4)  [unwired: 1 in]
      n52 = Get Date/Time String(seconds (now)=w142) -> (date string=w141:string, time string=w140:string)  [unwired: 2 in]
      n53 = Build Array(w141, w140) -> (w139:string[])
      "counter" <- w123
      "Path" <- w156
    }
    "A vs D" <- w39
    "C vs D" <- w40
    "time" <- w53
    "N Array" <- w20
    "A vs D diff" <- w19
    n54 = Transpose 2D Array(2D array=w38) -> (transposed array=w24:dbl[][])
    n55 = Transpose 2D Array(2D array=w37) -> (transposed array=w22:dbl[][])
    n56 = case shown="False" "calculate Ey" {
      tunnel: w31 -> [_ w79]
      tunnel: w30 -> [_ w78]
      tunnel: w29 -> [_ w67]
      tunnel: [w65 w74] -> w28
      tunnel: "Ey" -> [w65 _]
      frame False {
      }
      frame True {
        w70 = 2 items=["radian in, radian out", "radian in, degree out", "degree in, degree out", "degree in, radian out"] ("phase unit")
        n57 = Re/Im To Polar(2:w78, 3:w79) -> (0:w77:dbl[], 1:w66:dbl[])
        n58 = Re/Im To Polar(2:w66, 3:w67) -> (0:w68:dbl[])  [unwired: 1 out]
        n59 = expression code="x*180/pi"(w77) -> (w73:dbl[])
        n60 = expression code="x*180/pi"(w68) -> (w71:dbl[])
        n61 = call <userlib>:"OffsetMultiplier.vi"("Array"=w73) -> ("Offset"=w76:dbl, "Multiplier"=w75:dbl)
        n62 = call <vilib>:"Unwrap Phase.vi"("phase unit"=w70, "Phase"=w73) -> ("Unwrapped Phase"=→"angle theta":dbl[])  [unwired: 8 in, 1 out]
        n63 = call <vilib>:"Unwrap Phase.vi"("phase unit"=w70, "Phase"=w71) -> ("Unwrapped Phase"=→"angle phi":dbl[])  [unwired: 8 in, 1 out]
        n64 = Bundle("Offset"=w76, "Multiplier"=w75) -> (w74:cluster{"Offset":dbl, "Multiplier":dbl})  [unwired: 1 in]
      }
    }
    n65 = case shown="False" "log scale?" {
      tunnel: w24 -> [w60 w64]
      tunnel: [w60 w63] -> w23
      tunnel: w22 -> [w59 w62]
      tunnel: [w59 w61] -> w21
      frame False {
      }
      frame True {
        n66 = Logarithm Base 10(1:w64) -> (0:w63:dbl[][])
        n67 = Logarithm Base 10(1:w62) -> (0:w61:dbl[][])
      }
    }
    "E" <- w23
    "E 2" <- w21
    n68 = property on="E" class="IntGraph (strict)"("XScale.NameLbl.Text"="Ex name", "YScale.NameLbl.Text"="Ey name", "ZScale.NameLbl.Text"="Ez name") -> ()  [unwired: 2 in, 2 out]
    n69 = property on="E 2" class="IntGraph (strict)"("XScale.NameLbl.Text"="Ex name", "YScale.NameLbl.Text"="Ey name", "ZScale.NameLbl.Text"="Ez name") -> ()  [unwired: 2 in, 2 out]
    n70 = case shown="True" "recolor traces?" {
      tunnel: w39 -> [_ w80]
      frame False {
      }
      frame True {
        n71 = Array Size(array=w80) -> (size(s)=w83:i32)
        n72 = Reverse 1D Array(array=u32[] [16711680, 16772608, 6618880, 3381759, 16860, 10420479] ("color scale")) -> (reversed array=w82:u32[])
        n73 = Add(x=w83, y=0 ("x")) -> (x+y=w87:i32)
        n74 = call <userlib>:"Make Color Table.vi"("Array"=w82) -> ("Color Tbl"=w85:u32[])  [unwired: 1 in, 3 out]
        n75 = call <userlib>:"Make Color Table.vi"("Array"=w82, "Size/3"=w87) -> ("Color Tbl"=w84:u32[])  [unwired: 3 out]
        n76 = for {
          tunnel: w84 -> [w88] mode=indexing
          i -> [w89]
          n77 = property on="A vs D" class="XYGraph (strict)"("Active Plot"=w89, "Plot.Plot Color"=w88) -> (error out=w90:errorcluster)  [unwired: 2 in, 1 out]
          n78 = property on="C vs D" class="XYGraph (strict)"(error in=w90, "Active Plot"=w89, "Plot.Plot Color"=w88, "Plot.Fill/Pt. Color"=w88) -> ()  [unwired: 1 in, 2 out]
        }
        n79 = property on="E" class="IntGraph (strict)"("Color Table"=w85) -> ()  [unwired: 2 in, 2 out]
      }
    }
    n80 = property on="E" class="IntGraph (strict)"("XScale.Ofst&Mult"="Ex", "YScale.Ofst&Mult"=w28) -> ()  [unwired: 2 in, 2 out]
    n81 = property on="E 2" class="IntGraph (strict)"("XScale.Ofst&Mult"="Ex", "YScale.Ofst&Mult"="Ey") -> ()  [unwired: 2 in, 2 out]
    n82 = Select(t=7.0, s="D  is time?", f=8.0) -> (s? t:f=w45:dbl)
    n83 = Select(t=7.0, s="B is time?", f=8.0) -> (s? t:f=w46:dbl)
    n84 = property on="C vs D" class="XYGraph (strict)"("XScale.Format"=w45, "XScale.NameLbl.Text"="D x name", "YScale.NameLbl.Text"="C y name") -> ()  [unwired: 2 in, 2 out]
    n85 = property on="A vs D" class="XYGraph (strict)"("XScale.Format"=w46, "XScale.NameLbl.Text"="B x name", "YScale.NameLbl.Text"="A y name") -> ()  [unwired: 2 in, 2 out]
  }
